vi "CreateWarningMessagesToNotify.vi"(8 "IpStatus(in)":T2[](array[typedef]) {"%rtk" scale=0.0..60.0; "TimePing" scale=0.0..60.0}, 11 "IP list (in)":T1) -> (0 "IpStatus(out)":T2[](array[typedef]) {"%rtk" scale=0.0..60.0; "TimePing" scale=0.0..60.0}, 3 "IP list (out)":T1, 5 "Warning Messages":string[](array[string]), 7 "Send warnings":bool[](array[boolean]))   [LabVIEW 2011]
uses:
  GPS String Capture Software/IP RTK status Indicator.ctl
  ArrayIpAddressesAndReportingCheckbox.ctl
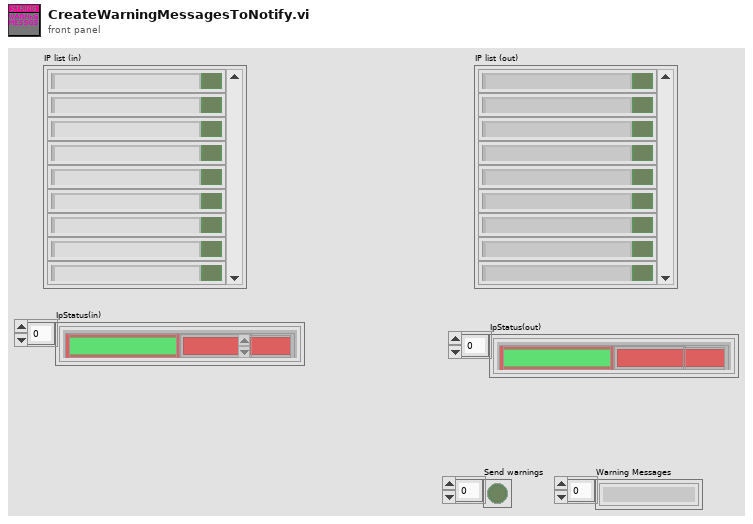
[diagram p1: front panel]
types:
  T1 = typedef "ArrayIpAddressesAndReportingCheckbox.ctl" = cluster{"IpAddress":string, "Report Errors":bool}[]
  T2 = typedef "IP RTK status Indicator.ctl" = cluster{"TimePing":dbl, "IP":string, "%rtk":dbl, "Lastrtk":string, "MinLastRTk":dbl, "RTK Count":bool[], "Last Nema Time":dbl, "Last RTK Time":dbl, "Last Ping time":dbl}
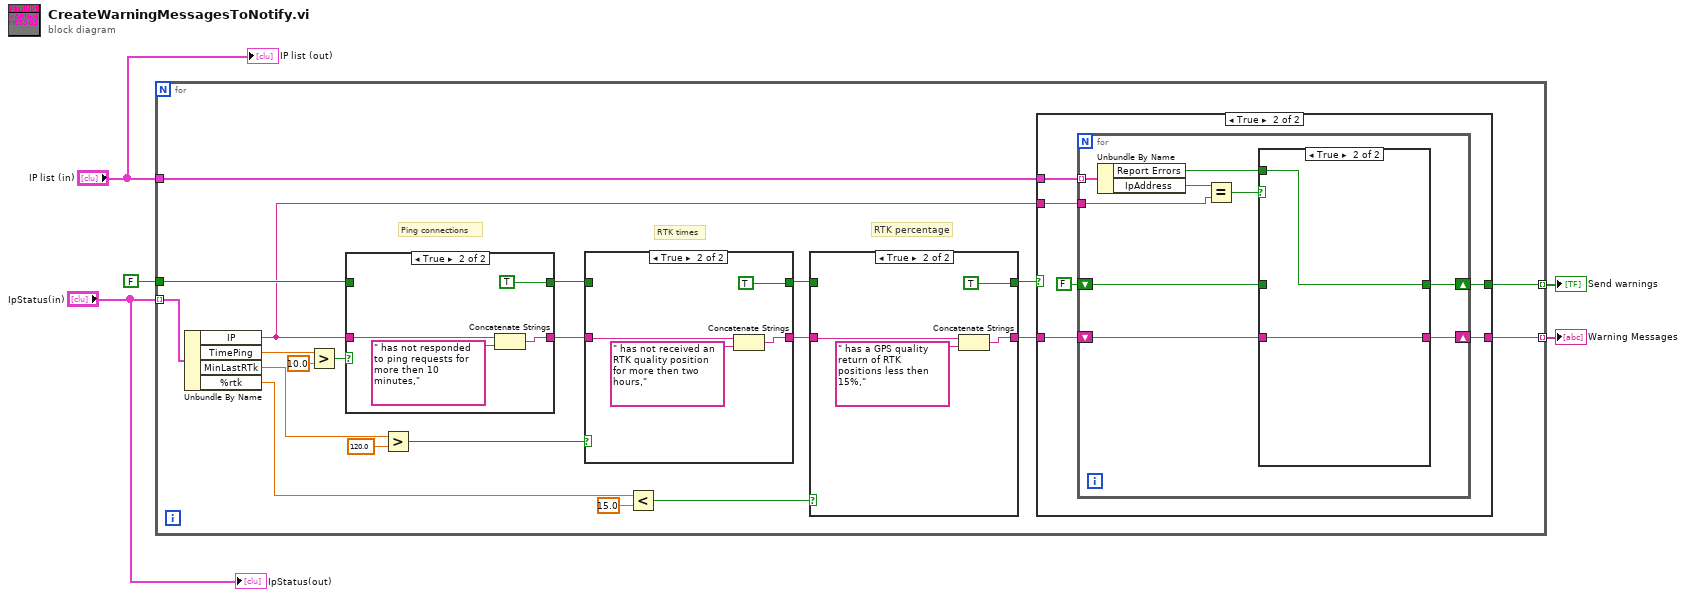
[diagram p0: block diagram]
diagram:
  n1 = for {
    tunnel: "IpStatus(in)" -> [w26] mode=indexing
    tunnel: FALSE -> [w22]
    tunnel: "IP list (in)" -> [w11]
    tunnel: [w7] -> w1 mode=indexing
    tunnel: [w6] -> w2 mode=indexing
    # "RTK percentage"
    # "RTK times"
    # "Ping connections"
    n2 = Unbundle By Name(w26) -> ("IP"=w8:string, "TimePing"=w25:dbl, "MinLastRTk"=w20:dbl, "%rtk"=w15:dbl)
    n3 = Greater?(x=w25, y=10.0) -> (0:w23:bool)
    n4 = case shown="True" w23 {
      tunnel: w22 -> [w61 _]
      tunnel: [w61 TRUE] -> w17
      tunnel: w8 -> [w60 w64]
      tunnel: [w60 w62] -> w19
      frame False {
      }
      frame True {
        n5 = Concatenate Strings(w64, " has not responded to ping requests for more then 10 minutes," ("string")) -> (w62:string)
      }
    }
    n6 = Greater?(x=w20, y=120.0) -> (0:w18:bool)
    n7 = case shown="True" w18 {
      tunnel: w17 -> [w55 _]
      tunnel: [w55 TRUE] -> w14
      tunnel: w19 -> [w54 w58]
      tunnel: [w54 w56] -> w13
      frame False {
      }
      frame True {
        n8 = Concatenate Strings(w58, " has not received an RTK quality position for more then two hours," ("string")) -> (w56:string)
      }
    }
    n9 = Less?(x=w15, y=15.0) -> (x < y?=w12:bool)
    n10 = case shown="True" w12 {
      tunnel: w14 -> [w49 _]
      tunnel: [w49 TRUE] -> w9
      tunnel: w13 -> [w48 w52]
      tunnel: [w48 w50] -> w10
      frame False {
      }
      frame True {
        n11 = Concatenate Strings(w52, " has a GPS quality return of RTK positions less then 15%," ("string")) -> (w50:string)
      }
    }
    n12 = case shown="True" w9 {
      selector: w9 -> [w27 _]
      tunnel: w11 -> [_ w34]
      tunnel: w10 -> [w28 w32]
      tunnel: w8 -> [_ w33]
      tunnel: [w28 w31] -> w7
      tunnel: [w27 w29] -> w6
      frame False {
      }
      frame True {
        n13 = for {
          tunnel: w34 -> [w43] mode=indexing
          tunnel: w33 -> [w41]
          shift-right: [w36] -> w31
          shift-left: w32 -> [w38]
          shift-right: [w37] -> w29
          shift-left: FALSE ("Report Errors") -> [w35]
          n14 = Unbundle By Name(w43) -> ("Report Errors"=w39:bool, "IpAddress"=w42:string)
          n15 = Equal?(x=w42, y=w41) -> (x = y?=w40:bool)
          n16 = case shown="True" w40 {
            tunnel: w39 -> [_ w47]
            tunnel: w38 -> [w45 w46]
            tunnel: [w44 w47] -> w37
            tunnel: [w45 w46] -> w36
            tunnel: w35 -> [w44 _]
            frame False {
            }
            frame True {
            }
          }
        }
      }
    }
  }
  "Send warnings" <- w2
  "Warning Messages" <- w1
  "IpStatus(out)" <- "IpStatus(in)"
  "IP list (out)" <- "IP list (in)"
